vi "Convert Amps-Tesla.vi"(3 "tesla":dbl, 5 "amps":dbl) -> (0 "ampsOUT":dbl, 2 "teslaOUT":dbl)   [LabVIEW 2023, in "Power Supply.lvclass"]
uses:
  Power Supply.lvclass
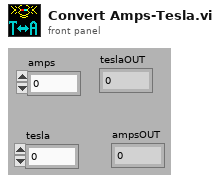
[diagram p1: front panel]
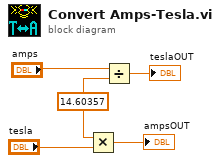
[diagram p0: block diagram]
diagram:
  w3 = 14.60357
  n1 = Multiply(x=w3, y="tesla") -> (x*y=→"ampsOUT":dbl)
  n2 = Divide(x="amps", y=w3) -> (x/y=→"teslaOUT":dbl)
